vi "LogAverage.vi"(10 "band power 2":dbl[](array[numeric]), 11 "band power":dbl[](array[numeric])) -> (3 "Array":dbl[](array[numeric]))   [LabVIEW 2017]
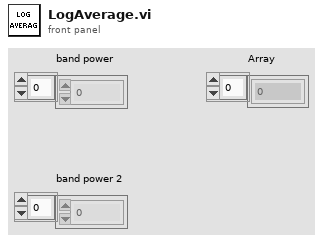
[diagram p1: front panel]
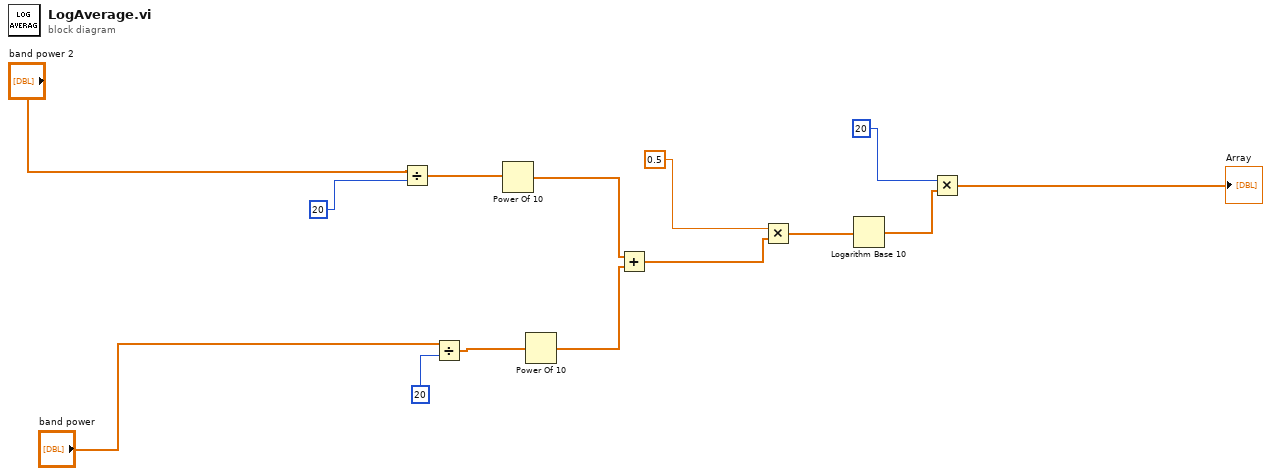
[diagram p0: block diagram]
diagram:
  n1 = Divide(x="band power 2", y=20) -> (x/y=w4:dbl[])
  n2 = Divide(x="band power", y=20) -> (x/y=w3:dbl[])
  n3 = Power Of 10(x=w4) -> (10^x=w5:dbl[])
  n4 = Power Of 10(x=w3) -> (10^x=w6:dbl[])
  n5 = Add(x=w5, y=w6) -> (x+y=w8:dbl[])
  n6 = Multiply(x=0.5, y=w8) -> (x*y=w9:dbl[])
  n7 = Logarithm Base 10(1:w9) -> (0:w11:dbl[])
  n8 = Multiply(x=20, y=w11) -> (x*y=→"Array":dbl[])
